vi "bezahlen.vi"() -> ()   [LabVIEW 2023]
panel:
  out "error out":errorcluster
  in  "error in (no error)":errorcluster
  out "Restgeldausgabe":dbl
  out "Betrag erreicht":bool
  in  "Storno":bool
  out "Guthaben":dbl
  in  "Preis":dbl
  in  "100 Euro":bool
  in  "50 Euro":bool
  in  "20 Euro":bool
  in  "10 Euro":bool
  in  "2 Euro":bool
  in  "5 Euro":bool
  in  "Bezahlen":bool
  in  "1 Euro":bool
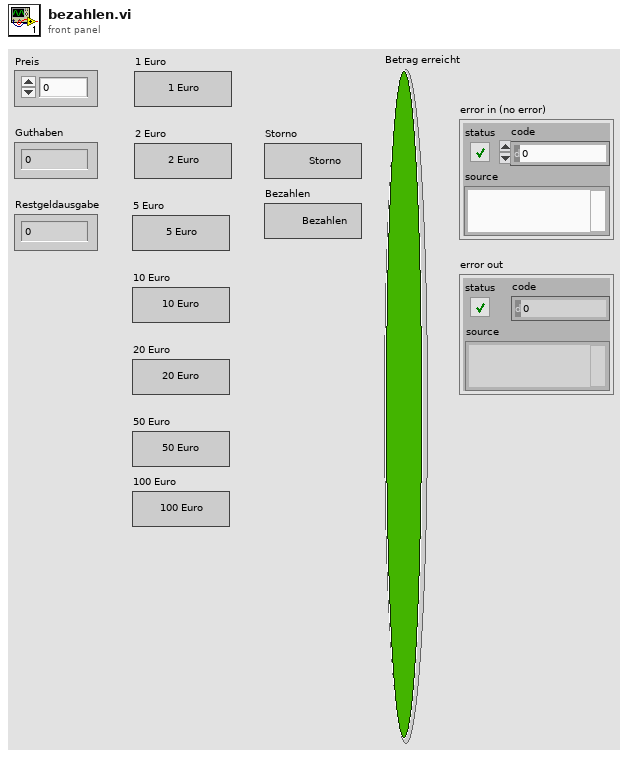
[diagram p1: front panel]
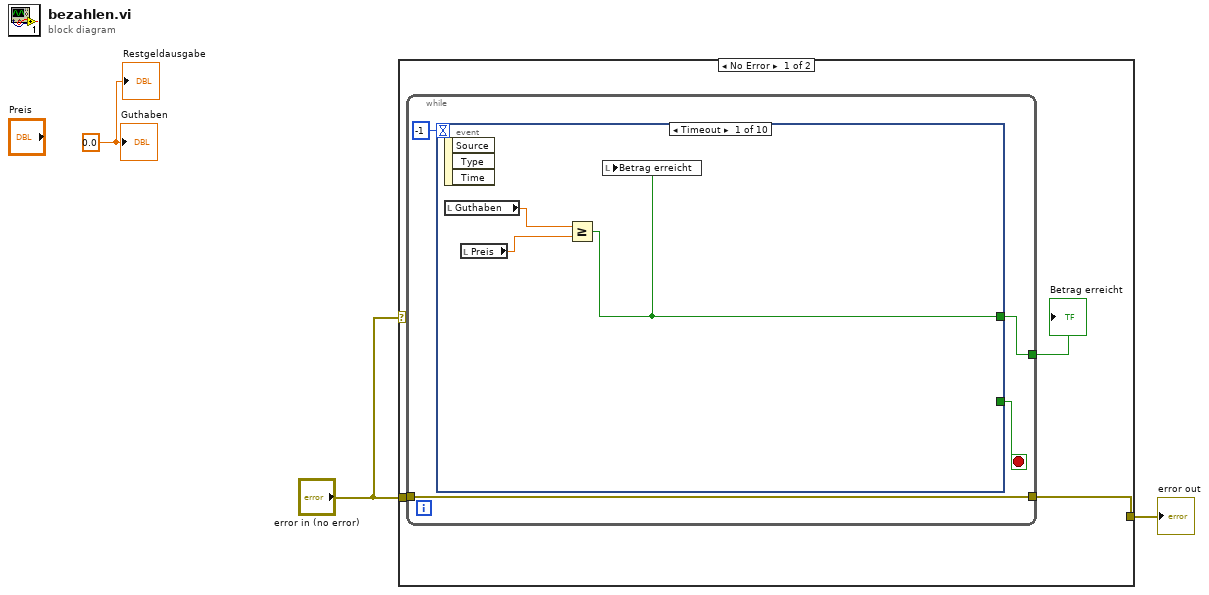
[diagram p0: block diagram]
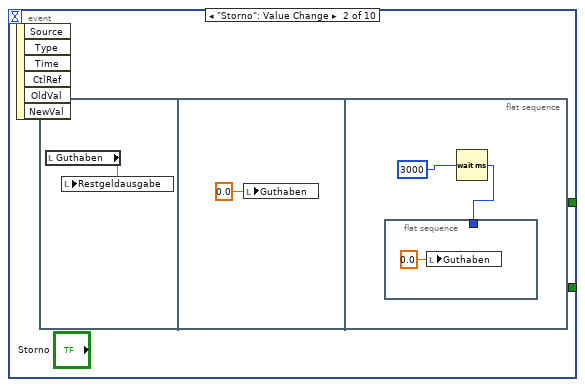
[diagram p2: hidden frame]
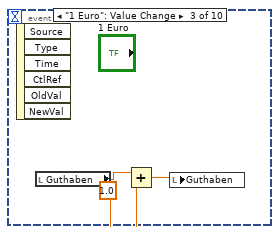
[diagram p3: hidden frame]
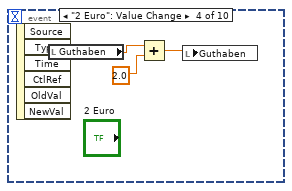
[diagram p4: hidden frame]
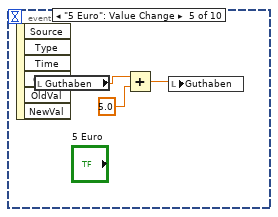
[diagram p5: hidden frame]
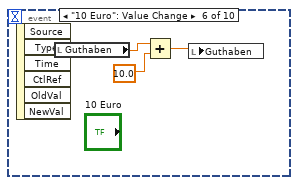
[diagram p6: hidden frame]
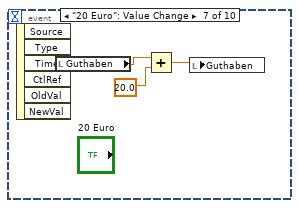
[diagram p7: hidden frame]
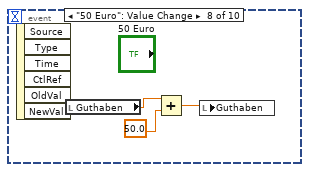
[diagram p8: hidden frame]
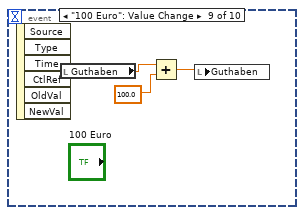
[diagram p9: hidden frame]
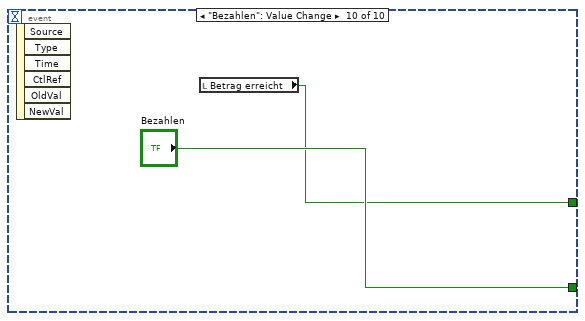
[diagram p10: hidden frame]
diagram:
  w3 = 0.0 ("Guthaben")
  n1 = case shown="No Error" "error in (no error)" {
    tunnel: "error in (no error)" -> [w6 w42]
    tunnel: [w5 w42] -> w2
    frame No Error {
      n2 = while {
        tunnel: [w9] -> w4
        tunnel: w6 -> [w8]
        tunnel: [w8] -> w5
        stop <- w10 stop-if-true
        n3 = event shown="[0] Timeout" {
          selector: _ -> [_ _ _ _ _ _ _ _ _ _]
          dyn-events: _ -> [_ _ _ _ _ _ _ _ _ _]
          timeout: -1 -> [_ _ _ _ _ _ _ _ _ _]
          tunnel: [_ _ _ _ _ _ _ _ _ "Bezahlen"] -> w10
          tunnel: [w11 _ _ _ _ _ _ _ _ w40] -> w9
          event Timeout {
            n4 = event-data() -> ()  [unwired: 1 in, 3 out]
            n5 = local read "Guthaben"() -> (w13:dbl)
            n6 = local read "Preis"() -> (w12:dbl)
            n7 = Greater Or Equal?(x=w13, y=w12) -> (x >= y?=w11:bool)
            n8 = local write "Betrag erreicht"(w11) -> ()
          }
          event "Storno": Value Change {
            n9 = event-data() -> ()  [unwired: 1 in, 6 out]
            n10 = flat-sequence {
              frame #0 {
                n11 = local read "Guthaben"() -> (w14:dbl)
                n12 = local write "Restgeldausgabe"(w14) -> ()
              }
              frame #1 {
                n13 = local write "Guthaben"(0.0 ("Guthaben")) -> ()
              }
              frame #2 {
                n14 = flat-sequence {
                  tunnel: w17 -> [_]
                  frame #0 {
                    n15 = local write "Guthaben"(0.0 ("Guthaben")) -> ()
                  }
                }
                n16 = Wait (ms)(milliseconds to wait=u32 3000 ("millisecond timer value")) -> (millisecond timer value=w17:u32)
              }
            }
          }
          event "1 Euro": Value Change {
            n17 = event-data() -> ()  [unwired: 1 in, 6 out]
            n18 = local read "Guthaben"() -> (w20:dbl)
            n19 = Add(x=w20, y=1.0) -> (x+y=w21:dbl)
            n20 = local write "Guthaben"(w21) -> ()
          }
          event "2 Euro": Value Change {
            n21 = event-data() -> ()  [unwired: 1 in, 6 out]
            n22 = local read "Guthaben"() -> (w23:dbl)
            n23 = Add(x=w23, y=2.0) -> (x+y=w24:dbl)
            n24 = local write "Guthaben"(w24) -> ()
          }
          event "5 Euro": Value Change {
            n25 = event-data() -> ()  [unwired: 1 in, 6 out]
            n26 = local read "Guthaben"() -> (w27:dbl)
            n27 = Add(x=w27, y=5.0) -> (x+y=w26:dbl)
            n28 = local write "Guthaben"(w26) -> ()
          }
          event "10 Euro": Value Change {
            n29 = event-data() -> ()  [unwired: 1 in, 6 out]
            n30 = local read "Guthaben"() -> (w28:dbl)
            n31 = Add(x=w28, y=10.0) -> (x+y=w30:dbl)
            n32 = local write "Guthaben"(w30) -> ()
          }
          event "20 Euro": Value Change {
            n33 = event-data() -> ()  [unwired: 1 in, 6 out]
            n34 = local read "Guthaben"() -> (w32:dbl)
            n35 = Add(x=w32, y=20.0) -> (x+y=w33:dbl)
            n36 = local write "Guthaben"(w33) -> ()
          }
          event "50 Euro": Value Change {
            n37 = event-data() -> ()  [unwired: 1 in, 6 out]
            n38 = local read "Guthaben"() -> (w35:dbl)
            n39 = Add(x=w35, y=50.0) -> (x+y=w36:dbl)
            n40 = local write "Guthaben"(w36) -> ()
          }
          event "100 Euro": Value Change {
            n41 = event-data() -> ()  [unwired: 1 in, 6 out]
            n42 = local read "Guthaben"() -> (w38:dbl)
            n43 = Add(x=w38, y=100.0) -> (x+y=w39:dbl)
            n44 = local write "Guthaben"(w39) -> ()
          }
          event "Bezahlen": Value Change {
            n45 = event-data() -> ()  [unwired: 1 in, 6 out]
            n46 = local read "Betrag erreicht"() -> (w40:bool)
          }
        }
      }
      "Betrag erreicht" <- w4
    }
    frame Error {
    }
  }
  "error out" <- w2
  "Guthaben" <- w3
  "Restgeldausgabe" <- w3
